vi "9602 Mandatory field missing for ObjectType--error.vi"(7 "Clear this Error?":bool, 8 "error in":errorcluster, 10 "Field Name":string, 11 "Object Type Base":refnum<class "Object Type Base.lvclass">) -> (0 "error out":errorcluster)   [LabVIEW 2019, in "Electronic Datasheet.lvlib"]
uses:
  Electronic Datasheet.lvlib
  Object Type/Object Type Base.lvclass
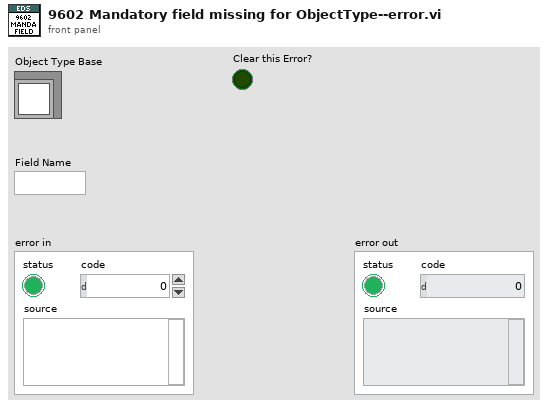
[diagram p1: front panel]
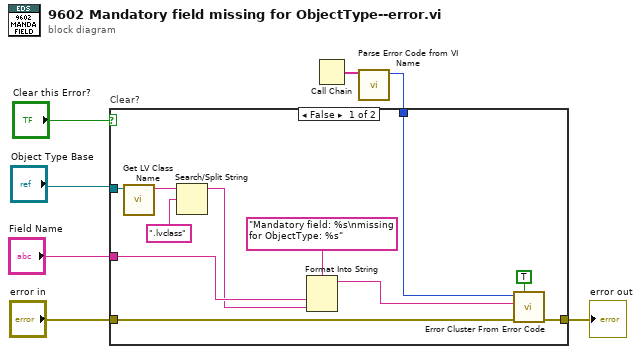
[diagram p0: block diagram]
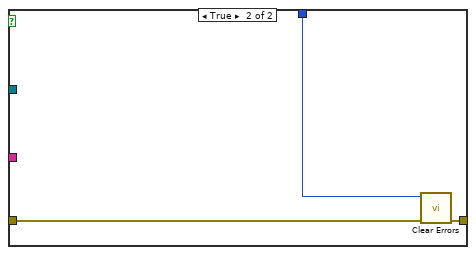
[diagram p2: hidden frame]
diagram:
  n1 = Call Chain() -> (call chain=w2:string[])
  n2 = call "Parse Error Code from VI Name.vi"("Call Chain"=w2) -> ("Error Code"=w1:i32)  [unwired: 10 in]
  n3 = case "Clear?" shown="False" "Clear this Error?" {
    tunnel: [w17 w20] -> w7
    tunnel: "Field Name" -> [w14 _]
    tunnel: "Object Type Base" -> [w13 _]
    tunnel: "error in" -> [w9 w21]
    tunnel: w1 -> [w8 w19]
    frame False {
      n4 = call <vilib>:"Get LV Class Name.vi"("object"=w13) -> ("class name"=w12:string)  [unwired: 9 in, 1 out]
      n5 = Search/Split String(string=w12, search string/char (-)=".lvclass") -> (substring before match=w10:string)  [unwired: 1 in, 2 out]
      n6 = Format Into String(format string="Mandatory field: %s\nmissing for ObjectType: %s", w14, w10) -> (resulting string=w15:string)  [unwired: 2 in, 1 out]
      n7 = call <vilib>:"Error Cluster From Error Code.vi"("show call chain? (False)"=TRUE, "error in (no error)"=w9, "error message (\"\")"=w15, "error code (0)"=w8) -> ("error out"=w17:errorcluster)  [unwired: 5 in]
    }
    frame True {
      n8 = call <vilib>:"Clear Errors.vi"("error in (no error)"=w21, "specific error code to clear (0: all)"=w19) -> ("error out"=w20:errorcluster)  [unwired: 4 in, 1 out]
    }
  }
  "error out" <- w7
